vi "SA5G_changeFrequency_NEW.vi"(5 "Enum":enum16{"Mark_Center_OFF", "Mark_Center_ON"}(ring), 7 "MHz":i32, 8 "error in":errorcluster, 11 "VISA in":refnum<visa-resource-name>) -> (0 "error out":errorcluster, 2 "SA_Resp":string, 3 "VISA out":refnum<visa-resource-name>)   [LabVIEW 2023, in "Keysight.lvlib"]
uses:
  Keysight.lvlib
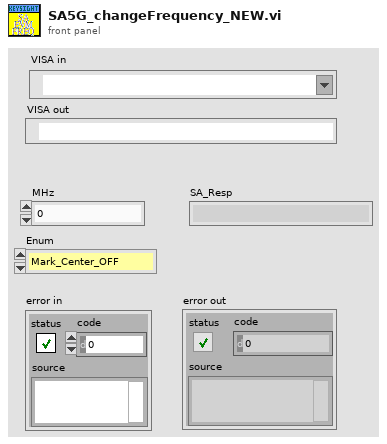
[diagram p1: front panel]
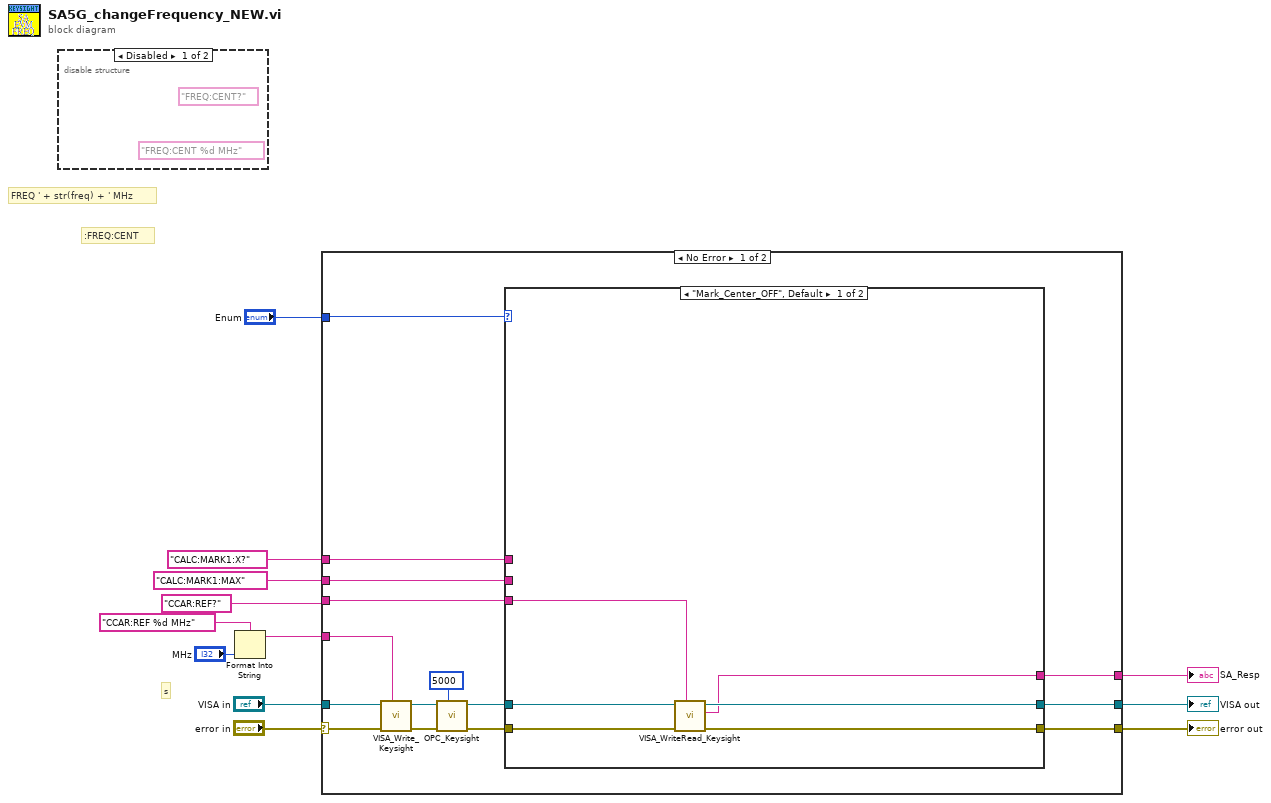
[diagram p0: block diagram]
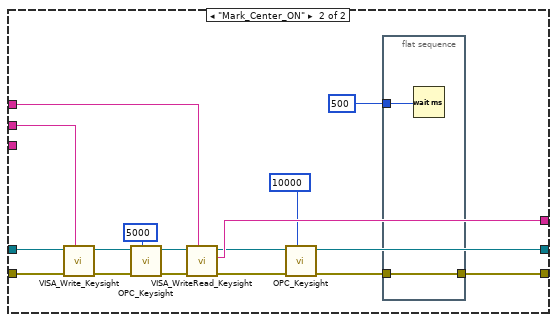
[diagram p3: hidden frame]
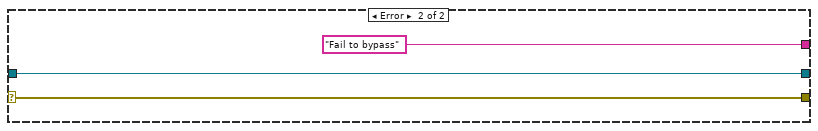
[diagram p4: hidden frame]
diagram:
  # ":FREQ:CENT"
  # "s"
  # "FREQ ' + str(freq) + ' MHz"
  n1 = disable-structure shown="Disabled" {
    frame Disabled {
      (unwired) "FREQ:CENT %d MHz" ("format string")
      (unwired) "FREQ:CENT?" ("write buffer")
    }
    frame Enabled {
    }
  }
  n2 = Format Into String(format string="CCAR:REF %d MHz", "MHz") -> (resulting string=w6:string)  [unwired: 2 in, 1 out]
  n3 = case shown="No Error" "error in" {
    selector: "error in" -> [w27 w54]
    tunnel: "VISA in" -> [w26 w55]
    tunnel: w6 -> [w25 _]
    tunnel: [w23 w54] -> w10
    tunnel: [w21 w55] -> w11
    tunnel: [w22 "Fail to bypass" ("Response")] -> w12
    tunnel: "CCAR:REF?" ("write buffer") -> [w14 _]
    tunnel: "Enum" -> [w24 _]
    tunnel: "CALC:MARK1:MAX" ("write buffer") -> [w20 _]
    tunnel: "CALC:MARK1:X?" ("write buffer") -> [w19 _]
    frame No Error {
      n4 = call "VISA_Write_Keysight.vi"("VISA CMD"=w25, "error in"=w27, "VISA in"=w26) -> ("error out"=w18:errorcluster, "VISA out"=w17:refnum<visa-resource-name>)  [unwired: 7 in]
      n5 = call "OPC_Keysight.vi"("Maximum Time (10000mSec)"=5000, "error in (no error)"=w18, "VISA resource name"=w17) -> ("error out"=w15:errorcluster, "VISA resource name out"=w16:refnum<visa-resource-name>)  [unwired: 7 in]
      n6 = case shown="\"Mark_Center_OFF\", Default" w24 {
        tunnel: w15 -> [w32 w50]
        tunnel: [w33 w35] -> w23
        tunnel: w16 -> [w30 w49]
        tunnel: [w28 w41] -> w22
        tunnel: [w31 w38] -> w21
        tunnel: w20 -> [_ w46]
        tunnel: w19 -> [_ w42]
        tunnel: w14 -> [w29 _]
        frame "Mark_Center_OFF", Default {
          n7 = call "VISA_WriteRead_Keysight.vi"("VISA_CMD"=w29, "error in"=w32, "VISA in"=w30) -> ("error out"=w33:errorcluster, "Response"=w28:string, "VISA out"=w31:refnum<visa-resource-name>)  [unwired: 6 in]
        }
        frame "Mark_Center_ON" {
          n8 = call "VISA_Write_Keysight.vi"("VISA CMD"=w46, "error in"=w50, "VISA in"=w49) -> ("error out"=w48:errorcluster, "VISA out"=w47:refnum<visa-resource-name>)  [unwired: 7 in]
          n9 = call "OPC_Keysight.vi"("Maximum Time (10000mSec)"=5000, "error in (no error)"=w48, "VISA resource name"=w47) -> ("error out"=w44:errorcluster, "VISA resource name out"=w43:refnum<visa-resource-name>)  [unwired: 7 in]
          n10 = call "VISA_WriteRead_Keysight.vi"("VISA_CMD"=w42, "error in"=w44, "VISA in"=w43) -> ("error out"=w37:errorcluster, "Response"=w41:string, "VISA out"=w39:refnum<visa-resource-name>)  [unwired: 6 in]
          n11 = call "OPC_Keysight.vi"("Maximum Time (10000mSec)"=10000, "error in (no error)"=w37, "VISA resource name"=w39) -> ("error out"=w36:errorcluster, "VISA resource name out"=w38:refnum<visa-resource-name>)  [unwired: 7 in]
          n12 = flat-sequence {
            tunnel: w36 -> [w52]
            tunnel: [w52] -> w35
            tunnel: u32 500 ("milliseconds to wait") -> [w51]
            frame #0 {
              n13 = Wait (ms)(milliseconds to wait=w51) -> ()  [unwired: 1 out]
            }
          }
        }
      }
    }
    frame Error {
    }
  }
  "SA_Resp" <- w12
  "VISA out" <- w11
  "error out" <- w10
